vi "GetErrorMsg.vi"(2 "ErrorCode":i32, 8 "error in (no error)":errorcluster) -> (0 "error out":errorcluster, 3 "ErrorMsg":string)   [LabVIEW 2022 SP3, in "EClib functions.lvlib"]
doc: "This VI stops loaded ecc protocols on the selected channel."
uses:
  EClib functions.lvlib
panel:
  out "errorcode":i32
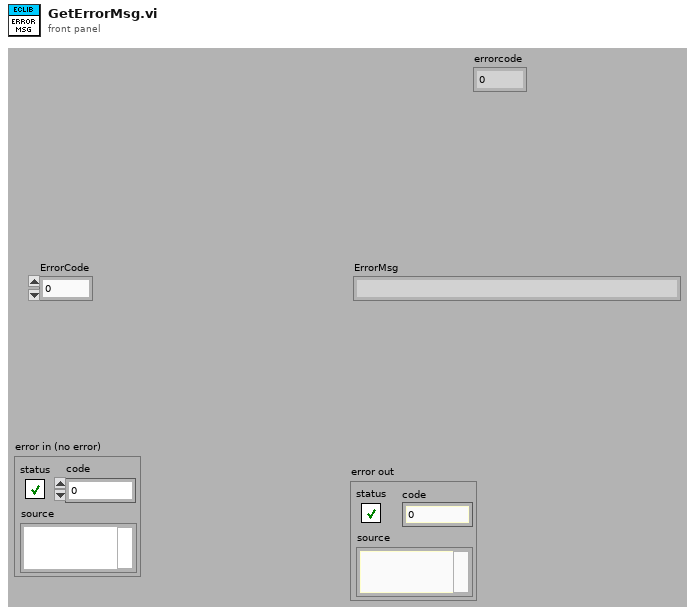
[diagram p1: front panel]
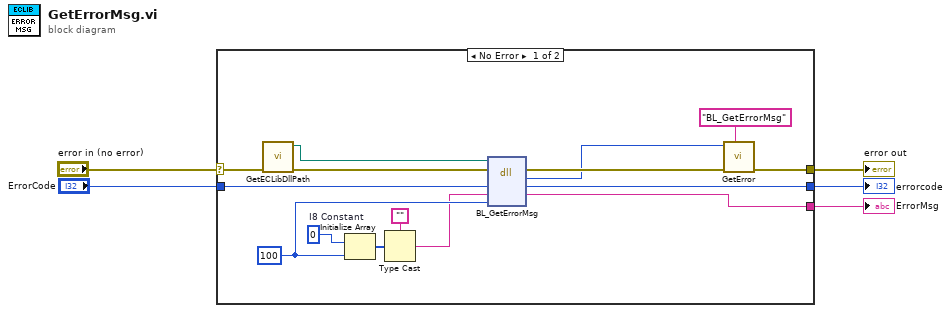
[diagram p0: block diagram]
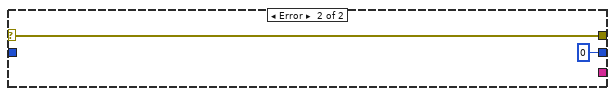
[diagram p2: hidden frame]
diagram:
  n1 = case shown="No Error" "error in (no error)" {
    selector: "error in (no error)" -> [w18 w22]
    tunnel: [w20 w22] -> w5
    tunnel: "ErrorCode" -> [w13 _]
    tunnel: [w12 _] -> w2
    tunnel: [w6 0 ("errorcode")] -> w1
    frame No Error {
      w11 = i8 0  # I8 Constant
      w8 = u32 100 ("psize")
      n2 = call "GetECLibDllPath.vi"("error in (no error)"=w18) -> ("error out"=w17:errorcluster, "ECLibDLLPath"=w14:path)  [unwired: 9 in]
      n3 = Initialize Array(w11, w8) -> (w10:i8[])
      n4 = Type Cast(type="", x=w10) -> (*(type *) &x=w7:string)
      n5 = dll-call lib="?" fn="BL_GetErrorMsg"(path in=w14, error in=w17, "errorcode"=w13, "pmsg"=w7, "psize"=w8) -> (error out=w16:errorcluster, "return type"=w15:i32, "errorcode"=w6:i32, "pmsg"=w12:string)  [unwired: 2 in, 1 out]
      n6 = call "GetError.vi"("DLLFunction"="BL_GetErrorMsg", "error in"=w16, "code"=w15) -> ("error out"=w20:errorcluster)  [unwired: 8 in]
    }
    frame Error {
    }
  }
  "error out" <- w5
  "ErrorMsg" <- w2
  "errorcode" <- w1
